vi "Set Item (JSON).vi"(8 "error in (no error)":errorcluster, 9 "JSON to Insert":string, 10 "Object (or Item) Path":string, 11 "CycloneDX SBOM in":refnum<class "CycloneDX JSON.lvclass">) -> (0 "error out":errorcluster, 3 "CycloneDX SBOM out":refnum<class "CycloneDX JSON.lvclass">)   [LabVIEW 2017, in "LabVIEW CycloneDX SBOM.lvlib" / "CycloneDX JSON.lvclass"]
doc: "Adds item (JSON) at the specified JSON path."
uses:
  CycloneDX JSON.lvclass
  CycloneDX JSON.lvclass/CycloneDX JSON.ctl
  <vilib>/JDP Science/JSONtext/JSONtext.lvlib
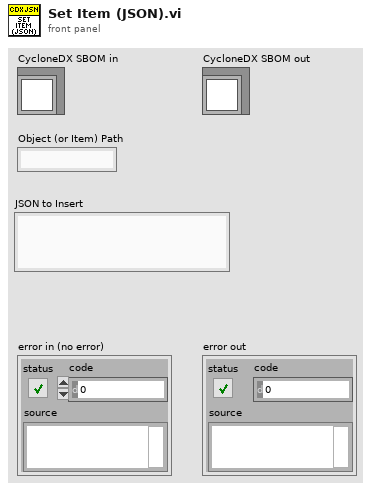
[diagram p1: front panel]
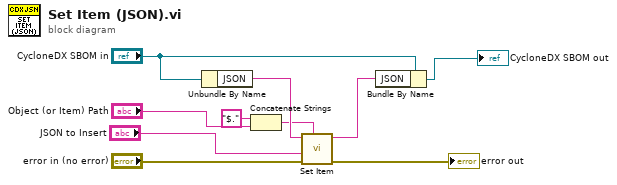
[diagram p0: block diagram]
diagram:
  n1 = Unbundle By Name("CycloneDX SBOM in") -> ("JSON"=w7:string)
  n2 = Concatenate Strings("$." ("string"), "Object (or Item) Path") -> (w1:string)
  n3 = call <vilib>:"Set Item.vi"("$Path or Item Name"=w1, "error in (no error)"="error in (no error)", "JSON to Insert"="JSON to Insert", "JSON"=w7) -> ("error out"=→"error out":errorcluster, "<JSON>"=w8:string)  [unwired: 4 in, 1 out]
  n4 = Bundle By Name(cluster="CycloneDX SBOM in", "JSON"=w8) -> (→"CycloneDX SBOM out":refnum<class "CycloneDX JSON.lvclass">)
